vi "SetPosition.vi"(8 "error in (no error)":errorcluster, 10 "position":cluster{"left":u32, "top":u32}, 11 "icon in":refnum<class "icon.lvclass">) -> (0 "error out":errorcluster, 3 "icon out":refnum<class "icon.lvclass">)   [LabVIEW 2009, in "icon.lvclass"]
uses:
  icon.lvclass
  icon.lvclass/icon.ctl
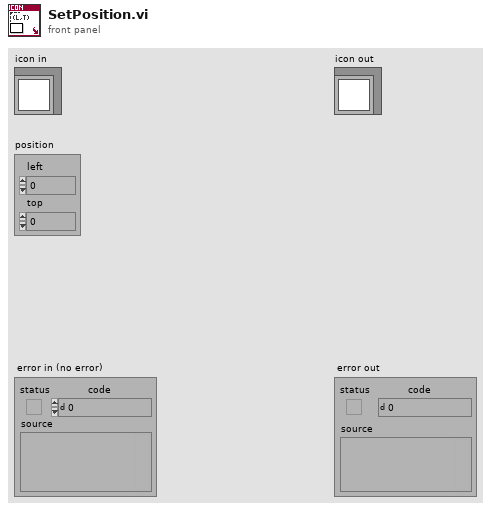
[diagram p1: front panel]
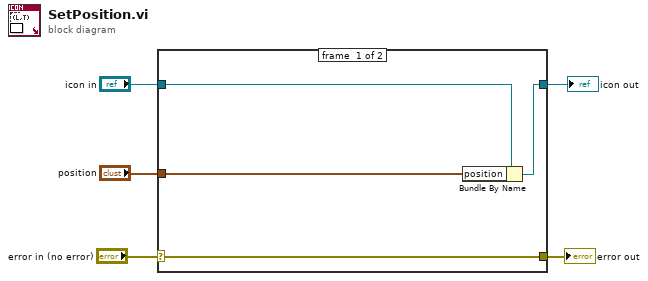
[diagram p0: block diagram]
diagram:
  n1 = case shown="No Error" "error in (no error)" {
    selector: "error in (no error)" -> [w9 w10]
    tunnel: [w9 w10] -> w2
    tunnel: [w7 w11] -> w4
    tunnel: "icon in" -> [w8 w11]
    tunnel: "position" -> [w6 _]
    frame #0 {
      n2 = Bundle By Name(cluster=w8, "position"=w6) -> (w7:refnum<class "icon.lvclass">)
    }
    frame #1 {
    }
  }
  "error out" <- w2
  "icon out" <- w4
